vi "PD500_Hydra - DC Bus Test_v1.vi"(11 "Board Selector":T1) -> (2 "INVB":dbl[](array[numeric]), 3 "INVA":dbl[](array[numeric]))   [LabVIEW 2022 SP3]
uses:
  Serial Board Com/Board Select.ctl
  HMP4000 Communication/HMP4040_ChannelControl.ctl
  Serial Board Com/ADCSelector GB.ctl
  Serial Board Com/ADCSelector BB.ctl
panel:
  in  "error in":errorcluster
  out "error out":errorcluster
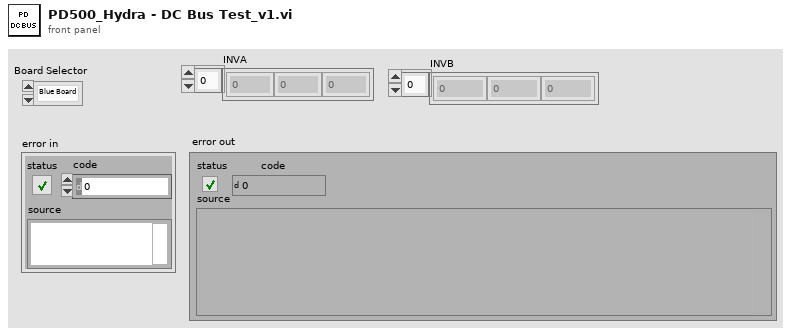
[diagram p1: front panel]
types:
  T1 = typedef "Board Select.ctl" = enum16{"Blue Board", "Green Board"}
  T2 = typedef "HMP4040_ChannelControl.ctl" = cluster{"CH1 Voltage":dbl, "CH1 Current":dbl, "CH1 Output":bool, "CH2 Voltage":dbl, "CH2 Current":dbl, "CH2 Output":bool, "CH3 Voltage":dbl, "CH3 Current":dbl, "CH3 Output":bool, "CH4 Voltage":dbl, "CH4 Current":dbl, "CH4 Output":bool, "Master Output":bool}
  T3 = cluster{"Relay Command":bool[], "Power Supply\nSettings":T2}[]
  T4 = typedef "ADCSelector BB.ctl" = enum16{"INVA_ISENSE_U", "INVA_ISENSE_V", "INVA_ISENSE_W", "INVA_UDC", "INVA_TEMP", "HB_TEMP", "AUXB_TEMP", "VLINE_AB", "VLINE_BC", "VLINE_CA", "VSENSE_POS_24V", "VSENSE_POS_5V", "VSENSE_NEG_15V", "INVB_ISENSE_U", "INV_B_ISENSEV", "INVB_ISENSE_W", "INVB_UDC", "INVB_TEMP", "AUXA_TEMP", "AUXC_TEMP", "VOUT_AB", "VOUT_BC", "VOUT_CA", "VSENSE_POS_15V", "VSENSE_POS_3P3V", "TEST_POINT"}
  T5 = typedef "ADCSelector GB.ctl" = enum16{"INVA_ISENSE_U", "INVA_ISENSE_V", "INVA_ISENSE_W", "INVA_UDC", "INVA_TEMP", "HB_ISENSE", "AUX_ISENSE_U", "AUX_ISENSE_V", "AUX_ISENSE_W", "VLINE_AB", "VLINE_BC", "VLINE_CA", "REF_1P5V", "VSENSE_POS_24V", "VSENSE_POS_5V", "VSENSE_NEG_15V", "TEST_POINT", "INVB_ISENSE_U", "INVB_ISENSE_V", "INVB_ISENSE_W", "INVB_UDC", "INVB_TEMP", "HB_TEMP", "AUXA_TEMP", "AUXB_TEMP", "AUXC_TEMP", "VOUT_AB", "VOUT_BC", "VOUT_CA", "REF_2P5V", "VSENSE_POS_15V", "VSENSE_POS_3P3V", "NET_ANALYZER"}
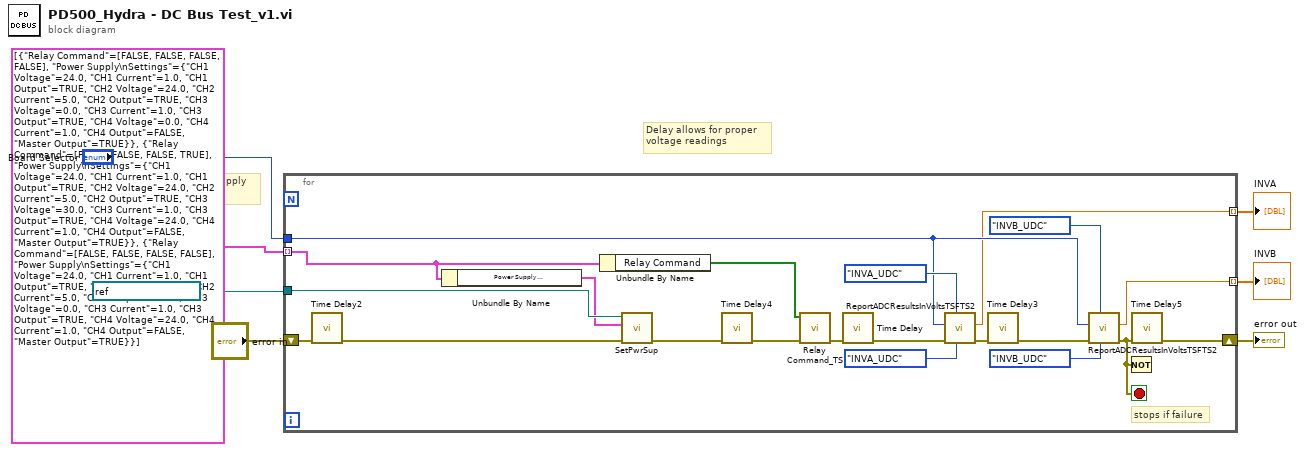
[diagram p0: block diagram]
diagram:
  # "Delay allows for proper \nvoltage readings"
  # "Settings for Power Supply\nand DC Contactor"
  n1 = for {
    shift-right: [w12] -> w7
    shift-left: "error in" -> [w22]
    tunnel: T3 [{"Relay Command"=[FALSE, FALSE, FALSE, FALSE], "Power Supply\nSettings"={"CH1 Voltage"=24.0, "CH1 Current"=1.0, "CH1 Output"=TRUE, "CH2 Voltage"=24.0, "CH2 Current"=5.0, "CH2 Output"=TRUE, "CH3 Voltage"=0.0, "CH3 Current"=1.0, "CH3 Output"=TRUE, "CH4 Voltage"=0.0, "CH4 Current"=1.0, "CH4 Output"=FALSE, "Master Output"=TRUE}}, {"Relay Command"=[FALSE, FALSE, FALSE, TRUE], "Power Supply\nSettings"={"CH1 Voltage"=24.0, "CH1 Current"=1.0, "CH1 Output"=TRUE, "CH2 Voltage"=24.0, "CH2 Current"=5.0, "CH2 Output"=TRUE, "CH3 Voltage"=30.0, "CH3 Current"=1.0, "CH3 Output"=TRUE, "CH4 Voltage"=24.0, "CH4 Current"=1.0, "CH4 Output"=FALSE, "Master Output"=TRUE}}, {"Relay Command"=[FALSE, FALSE, FALSE, FALSE], "Power Supply\nSettings"={"CH1 Voltage"=24.0, "CH1 Current"=1.0, "CH1 Output"=TRUE, "CH2 Voltage"=24.0, "CH2 Current"=5.0, "CH2 Output"=TRUE, "CH3 Voltage"=0.0, "CH3 Current"=1.0, "CH3 Output"=TRUE, "CH4 Voltage"=24.0, "CH4 Current"=1.0, "CH4 Output"=FALSE, "Master Output"=TRUE}}] -> [w26] mode=indexing
    tunnel: "Board Selector" -> [w23]
    tunnel: [w20] -> w5 mode=indexing
    tunnel: [w19] -> w4 mode=indexing
    tunnel: refnum<visa-resource-name> "HMP4040_FTS2" ("HMP4040 IN") -> [w11]
    stop <- w13 stop-if-true
    # "stops if failure"
    n2 = call "Time Delay2"("error in (no error)"=w22) -> ("error out"=w9:errorcluster)  [unwired: 10 in]
    n3 = Unbundle By Name(w26) -> ("Power Supply\nSettings"=w10:T2)
    n4 = Unbundle By Name(w26) -> ("Relay Command"=w21:bool[])
    n5 = call "SetPwrSup.vi"("error in (no error)"=w9, "HMP4040 Channel Settings"=w10, "HMP4040 IN"=w11) -> ("error out"=w8:errorcluster)  [unwired: 7 in, 1 out]
    n6 = call "Time Delay4"("error in (no error)"=w8) -> ("error out"=w14:errorcluster)  [unwired: 10 in]
    n7 = call "Relay Command_TS.vi"("error in (no error)"=w14, "Relay Command"=w21) -> ("error out"=w27:errorcluster)  [unwired: 8 in, 1 out]
    n8 = call "Time Delay"("error in (no error)"=w27) -> ("error out"=w28:errorcluster)  [unwired: 10 in]
    n9 = call "ReportADCResultsInVoltsTSFTS2.vi"("Blue Board Enum"=ADCSelector_BB."INVA_UDC", "Green Board Enum"=ADCSelector_GB."INVA_UDC" ("Enum"), "error in (no error)"=w28, "Board Selector"=w23) -> ("error out"=w16:errorcluster, "Result"=w20:dbl)  [unwired: 4 in, 2 out]
    n10 = call "Time Delay3"("error in (no error)"=w16) -> ("error out"=w15:errorcluster)  [unwired: 10 in]
    n11 = call "ReportADCResultsInVoltsTSFTS2.vi"("Blue Board Enum"=ADCSelector_BB."INVB_UDC", "Green Board Enum"=ADCSelector_GB."INVB_UDC" ("Enum"), "error in (no error)"=w15, "Board Selector"=w23) -> ("error out"=w13:errorcluster, "Result"=w19:dbl)  [unwired: 4 in, 2 out]
    n12 = Not(x=w13) -> ()  [unwired: 1 out]
    n13 = call "Time Delay5"("error in (no error)"=w13) -> ("error out"=w12:errorcluster)  [unwired: 10 in]
  }
  "error out" <- w7
  "INVA" <- w5
  "INVB" <- w4
